vi "History Update for Spartan 5.0.vi"(8 "error in (no error)":errorcluster, 10 "Old History Record":T1) -> (0 "error out":errorcluster, 2 "New History Record":T1)   [LabVIEW 2011]
uses:
  History Record.ctl
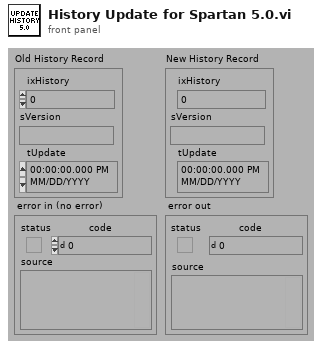
[diagram p1: front panel]
types:
  T1 = typedef "History Record.ctl" = cluster{"ixHistory":i32, "sVersion":string, "tUpdate":timestamp}
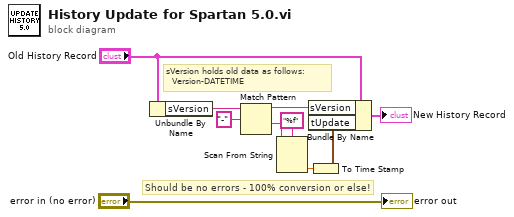
[diagram p0: block diagram]
diagram:
  # "sVersion holds old data as follows:\n  Version-DATETIME"
  # "Should be no errors - 100% conversion or else!"
  n1 = Unbundle By Name("Old History Record") -> ("sVersion"=w5:string)
  n2 = Match Pattern(string=w5, regular expression="-") -> (before substring=w3:string, after substring=w6:string)  [unwired: 3 out]
  n3 = Scan From String(format string="%f", input string=w6) -> (output 1=w2:dbl)  [unwired: 2 in, 4 out]
  n4 = To Time Stamp(1:w2) -> (0:w1:timestamp)
  n5 = Bundle By Name(cluster="Old History Record", "sVersion"=w3, "tUpdate"=w1) -> (→"New History Record":T1)
  "error out" <- "error in (no error)"
